vi "LeastDistantAngle.vi"(3 "Enum":enum16{"within pi", "within pi/2"}(ring)=enum."within pi/2", 4 "Current angle":dbl, 5 "target angle (between pi and -pi)":dbl(knob) scale=3.14159..-3.14159) -> (0 "current angle (between pi and -pi)":dbl(knob) scale=3.14159..-3.14159, 1 "Reverse?":bool, 2 "output angle":dbl)   [LabVIEW 2015]
panel:
  out "within pi":dbl(knob) scale=3.14159..-3.14159
  out "within pi/2":dbl(knob) scale=3.14159..-3.14159
  out "straightforward delta":dbl(knob) scale=3.14159..-3.14159
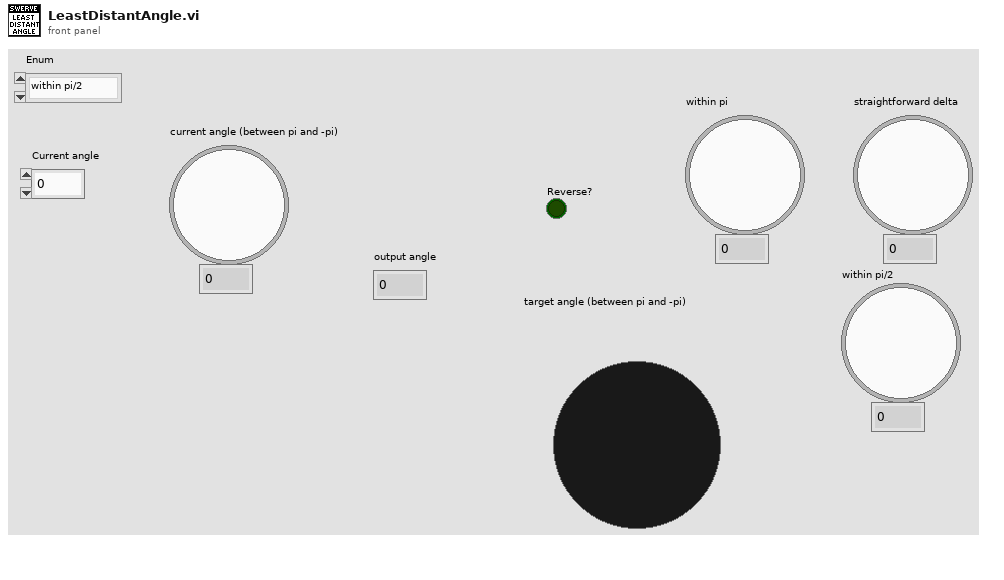
[diagram p1: front panel]
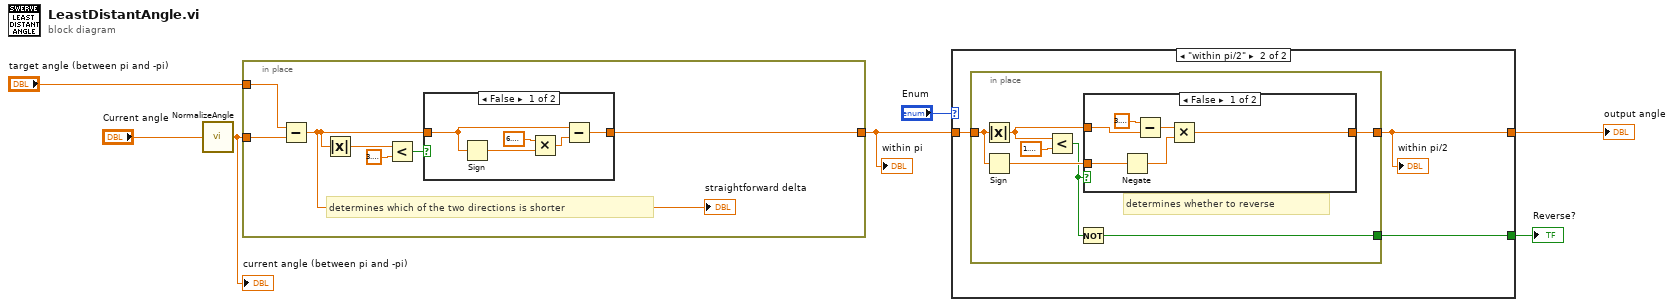
[diagram p0: block diagram]
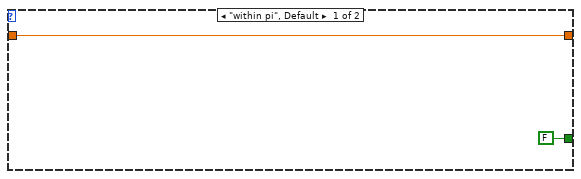
[diagram p2: hidden frame]
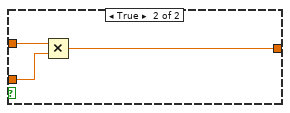
[diagram p3: hidden frame]
diagram:
  n1 = call "NormalizeAngle.vi"("angle (rad)"="Current angle") -> ("angle (between pi and -pi)"=w2:dbl)
  "current angle (between pi and -pi)" <- w2
  n2 = in-place {
    in-place-border: "target angle (between pi and -pi)" -> [w10]
    in-place-border: w2 -> [w9]
    in-place-border: [w11] -> w7
    # "determines which of the two directions is shorter"
    n3 = Subtract(x=w10, y=w9) -> (x-y=w8:dbl)
    "straightforward delta" <- w8
    n4 = Absolute Value(x=w8) -> (abs(x)=w14:dbl)
    n5 = Less?(x=w14, y=3.141592653589793) -> (x < y?=w13:bool)
    n6 = case shown="False" w13 {
      tunnel: w8 -> [w16 w20]
      tunnel: [w15 w20] -> w11
      frame False {
        n7 = Sign(1:w16) -> (0:w18:dbl)
        n8 = Multiply(x=6.283185307179586, y=w18) -> (x*y=w17:dbl)
        n9 = Subtract(x=w16, y=w17) -> (x-y=w15:dbl)
      }
      frame True {
      }
    }
  }
  "within pi" <- w7
  n10 = case shown="\"within pi/2\"" "Enum" {
    tunnel: w7 -> [w22 w25]
    tunnel: [w22 w23] -> w1
    tunnel: [FALSE w24] -> w5
    frame "within pi", Default {
    }
    frame "within pi/2" {
      n11 = in-place {
        in-place-border: w25 -> [w32]
        in-place-border: [w28] -> w23
        in-place-border: [w26] -> w24
        # "determines whether to reverse"
        n12 = Absolute Value(x=w32) -> (abs(x)=w29:dbl)
        n13 = Sign(1:w32) -> (0:w30:dbl)
        n14 = Less?(x=w29, y=1.5707963267948966) -> (x < y?=w27:bool)
        n15 = Not(x=w27) -> (.not. x?=w26:bool)
        n16 = case shown="False" w27 {
          tunnel: w30 -> [w35 w40]
          tunnel: w29 -> [w38 w41]
          tunnel: [w34 w39] -> w28
          frame False {
            n17 = Negate(x=w35) -> (-x=w33:dbl)
            n18 = Subtract(x=3.141592653589793, y=w38) -> (x-y=w36:dbl)
            n19 = Multiply(x=w36, y=w33) -> (x*y=w34:dbl)
          }
          frame True {
            n20 = Multiply(x=w41, y=w40) -> (x*y=w39:dbl)
          }
        }
      }
      "within pi/2" <- w23
    }
  }
  "output angle" <- w1
  "Reverse?" <- w5
